vi "Save scan settings.vi"(8 "Path":path, 10 "New scan settings":T1={"J-V scan"=TRUE, "J-t scan"=FALSE, "Min voltage (V)"=0.0, "Max voltage (V)"=1.4, "Step (V)"=0.01, "Measurement delay (ms)"=10.0, "1st scan FB-SC"=TRUE, "Inverted structure"=FALSE, "Stabilisation time (s)"=0.0, "Stabilisation mode"=0, "Stabilisation value (V or A) "=0.0, "Step time (s)"=1.0, "Integration time"=0, "Repeat light scans"=FALSE, "Stabilisation in the dark?"=FALSE, "J-t Min (V)"=0.0, "J-t Max (V)"=1.4, "J-t Step (V)"=0.01, "Max. power stabilisation"=FALSE, "J-t 1st scan FB-SC"=TRUE, "J-t Inverted structure"=FALSE, "Max power tracking"=FALSE, "Vmp (V)"=0.7, "Total stabilisation time (s)"=100.0, "J-t best pixel only"=0, "Max power best pixel only"=0, "Vmp from J-V scan"=FALSE, "Intensity dependence"=FALSE, "P dep best pixel only"=0, "External quantum efficiency"=FALSE, "EQE best pixel only"=0, "WL min (nm)"=300.0, "WL max (nm)"=900.0, "WL step (nm)"=5.0, "Wait (ms)"=100.0, "No. of repeat scans"=2.0, "Only repeat for best pixel"=0, "Chopper Freq.  (Hz)"=90.0, "Time Constant (s)"=2.0, "Stabilisation time step (s)"=1.0, "Illumination conditions"=2, "Scan rate min (V/s)"=0.1, "Scan rate max (V/s)"=1.0, "No. of scan rate steps"=1.0, "Scan rate voltage step priority"=FALSE, "Scan rate measurement delay priority"=FALSE, "J-t Illumination conditions"=0, "White bias  (no. of suns)"=200.0, "Max P stab. Specific voltage"=FALSE} {"J-t Illumination conditions" items=["Light only", "Dark only", "Light then dark", "Dark then light"]; "No. of scan rate steps" min=1.0 step=1.0; "Illumination conditions" items=["Light only", "Dark only", "Light then dark", "Dark then light", "Light then dark then light", "Dark then light then dark"]; "Time Constant (s)" items=["0.01s", "0.03s", "0.1s", "0.3s", "1s", "3s"]; "Only repeat for best pixel" items=["only for best pixel", "for best 2 pixels", "for best 3 pixels", "for best 4 pixels", "for best 5 pixels", "for best 6 pixels", "for best 7 pixels", "for all pixels"]; "No. of repeat scans" min=1.0 step=1.0; "EQE best pixel only" items=["only the best pixel", "the best 2 pixel", "the best 3 pixel", "the best 4 pixel", "the best 5 pixel", "the best 6 pixel", "the best 7 pixel", "all pixels"]; "P dep best pixel only" items=["only the best pixel", "the best 2 pixels", "the best 3 pixels", "the best 4 pixels", "the best 5 pixels", "the best 6 pixels", "the best 7 pixels", "all pixels"]; "Max power best pixel only" items=["only the best pixel", "the best 2 pixels", "the best 3 pixels", "the best 4 pixels", "the best 5 pixels", "the best 6 pixels", "the best 7 pixels", "all pixels"]; "J-t best pixel only" items=["only the best pixel", "the best 2 pixels", "the best 3 pixels", "the best 4 pixels", "the best 5 pixels", "the best 6 pixels", "the best 7 pixels", "all pixels"]; "Integration time" items=["Fast", "Normal", "High Accuracy"]; "Stabilisation mode" items=["V", "I"]; "Measurement delay (ms)" min=10.0}, 11 "New name":string) -> (0 "error out":errorcluster)   [LabVIEW 2011]
uses:
  TypeDefs/Scan settings.ctl
  TypeDefs/Settings Boolean.ctl
  <vilib>/Utility/file.llb/Write To Spreadsheet File (string).vi
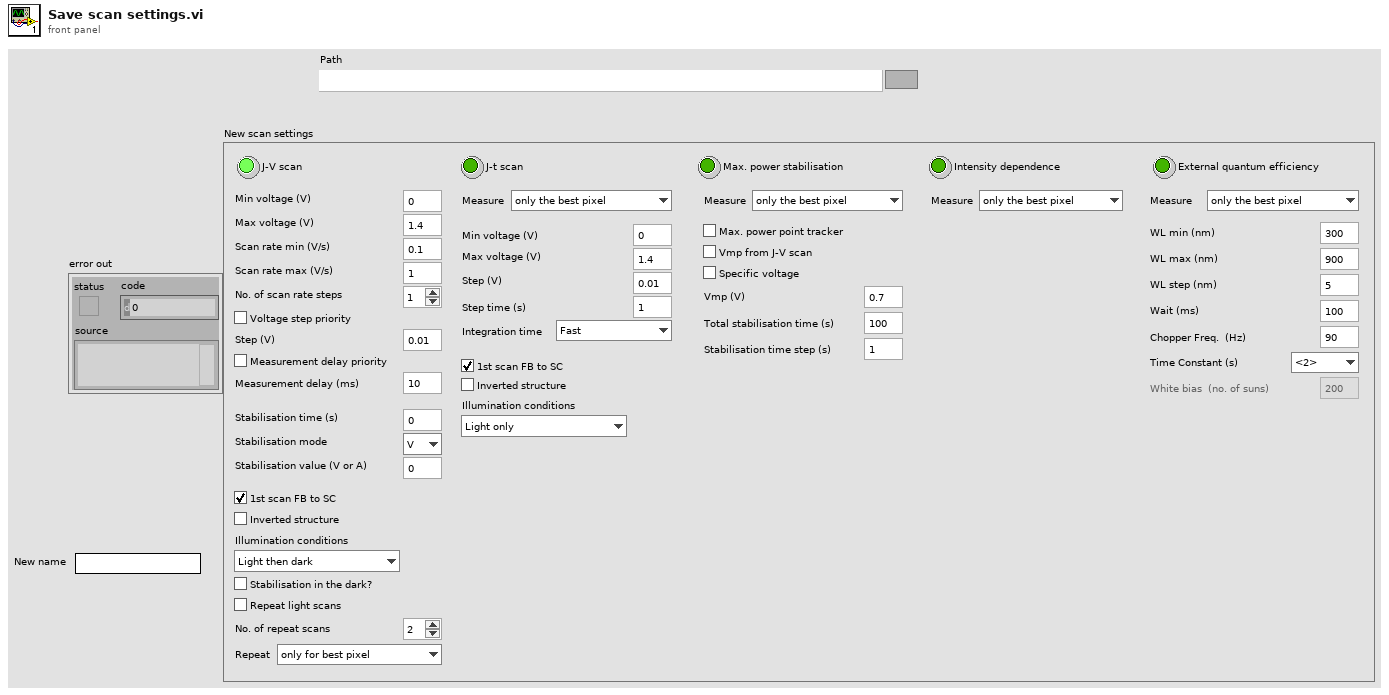
[diagram p1: front panel]
types:
  T1 = typedef "Scan settings.ctl" = cluster{"J-V scan":T2, "J-t scan":bool, "Min voltage (V)":dbl, "Max voltage (V)":dbl, "Step (V)":dbl, "Measurement delay (ms)":dbl, "1st scan FB-SC":bool, "Inverted structure":bool, "Stabilisation time (s)":dbl, "Stabilisation mode":u16, "Stabilisation value (V or A) ":dbl, "Step time (s)":dbl, "Integration time":u16, "Repeat light scans":bool, "Stabilisation in the dark?":bool, "J-t Min (V)":dbl, "J-t Max (V)":dbl, "J-t Step (V)":dbl, "Max. power stabilisation":bool, "J-t 1st scan FB-SC":bool, "J-t Inverted structure":bool, "Max power tracking":bool, "Vmp (V)":dbl, "Total stabilisation time (s)":dbl, "J-t best pixel only":u16, "Max power best pixel only":u16, "Vmp from J-V scan":bool, "Intensity dependence":bool, "P dep best pixel only":u16, "External quantum efficiency":bool, "EQE best pixel only":u16, "WL min (nm)":dbl, "WL max (nm)":dbl, "WL step (nm)":dbl, "Wait (ms)":dbl, "No. of repeat scans":dbl, "Only repeat for best pixel":u16, "Chopper Freq.  (Hz)":dbl, "Time Constant (s)":dbl, "Stabilisation time step (s)":dbl, "Illumination conditions":u16, "Scan rate min (V/s)":dbl, "Scan rate max (V/s)":dbl, "No. of scan rate steps":dbl, "Scan rate voltage step priority":bool, "Scan rate measurement delay priority":bool, "J-t Illumination conditions":u16, "White bias  (no. of suns)":dbl, "Max P stab. Specific voltage":bool}
  T2 = typedef "Settings Boolean.ctl" = bool
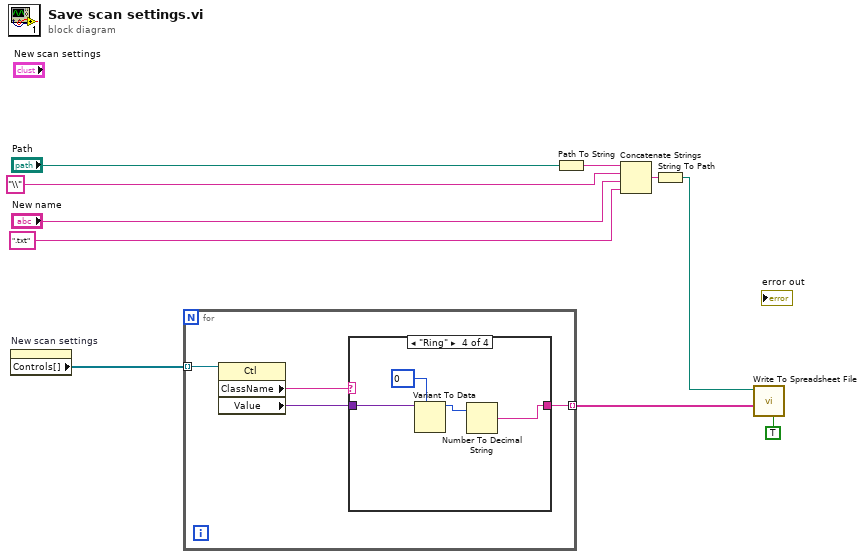
[diagram p0: block diagram]
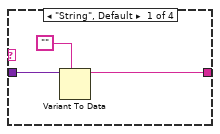
[diagram p2: hidden frame]
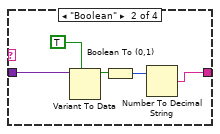
[diagram p3: hidden frame]
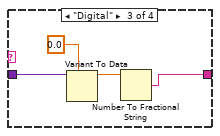
[diagram p4: hidden frame]
diagram:
  n1 = property on="New scan settings" class="Clust (strict)"() -> ("Controls[]"=w4:refnum<vi>[])  [unwired: 2 in, 2 out]
  n2 = for {
    tunnel: w4 -> [w14] mode=indexing
    tunnel: [w11] -> w2 mode=indexing
    n3 = property class="Ctl"(reference=w14) -> ("ClassName"=w13:string, "Value"=w12:variant)  [unwired: 1 in, 2 out]
    n4 = case shown="\"Ring\"" w13 {
      tunnel: w12 -> [w17 w22 w26 w28]
      tunnel: [w15 w18 w23 w27] -> w11
      frame "String", Default {
        n5 = Variant To Data(type="", Variant=w17) -> (data=w15:string)  [unwired: 1 in, 1 out]
      }
      frame "Boolean" {
        n6 = Variant To Data(type=TRUE, Variant=w22) -> (data=w20:bool)  [unwired: 1 in, 1 out]
        n7 = Boolean To (0,1)(Boolean=w20) -> (0, 1=w19:i16)
        n8 = Number To Decimal String(number=w19) -> (decimal integer string=w18:string)  [unwired: 1 in]
      }
      frame "Digital" {
        n9 = Variant To Data(type=0.0, Variant=w26) -> (data=w24:dbl)  [unwired: 1 in, 1 out]
        n10 = Number To Fractional String(number=w24) -> (F-format string=w23:string)  [unwired: 3 in]
      }
      frame "Ring" {
        w30 = u16 0 items=[""]
        n11 = Variant To Data(type=w30, Variant=w28) -> (data=w29:u16)  [unwired: 1 in, 1 out]
        n12 = Number To Decimal String(number=w29) -> (decimal integer string=w27:string)  [unwired: 1 in]
      }
    }
  }
  n13 = Path To String(path="Path") -> (string=w10:string)
  n14 = Concatenate Strings(w10, "\\", "New name", ".txt" ("y")) -> (w9:string)
  n15 = String To Path(string=w9) -> (path=w3:path)
  n16 = call-poly <vilib>:"Write To Spreadsheet File.vi"("transpose? (no:F)"=TRUE, "1D data"=w2, "file path (dialog if empty)"=w3) -> ()  [unwired: 5 in, 1 out]
